vi "Execute Path with commands.vi"(0 "Iterations":i32, 1 "Sample Period":dbl, 2 "Commands":T2(array[cluster]) {"System" items=["Elevator", "Floating Intake", "Carriage Intake"]; "System Selection" items=["Elevator", "Floating Intake", "Carriage Intake"]}) -> ()   [LabVIEW 2018]
doc: "This VI notifies the subsystem to the new setpoint."
uses:
  Availible Command systems for auto.ctl
  <vilib>/Rock Robotics/WPI/Framework/Command Status Info.ctl
  <vilib>/Rock Robotics/WPI/Framework/Completion Status.ctl
  <vilib>/Rock Robotics/WPI/Framework/Completion Notifier.ctl
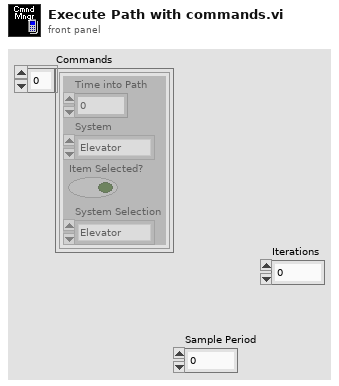
[diagram p1: front panel]
types:
  T1 = typedef "Availible Command systems for auto.ctl" = u16
  T2 = cluster{"Time into Path":dbl, "System":T1, "Item Selected?":bool, "System Selection":T1}[]
  T3 = cluster{"Time into Path":dbl, "System":T1, "Item Selected?":bool, "System Selection":T1}
  T4 = typedef "Command Status Info.ctl" = cluster{"Name":string, "Status":T5, "notifier out":T6}
  T5 = typedef "Completion Status.ctl" = enum16{"Successful", "Aborted", "Incomplete"}
  T6 = typedef "Completion Notifier.ctl" = refnum<notifier>
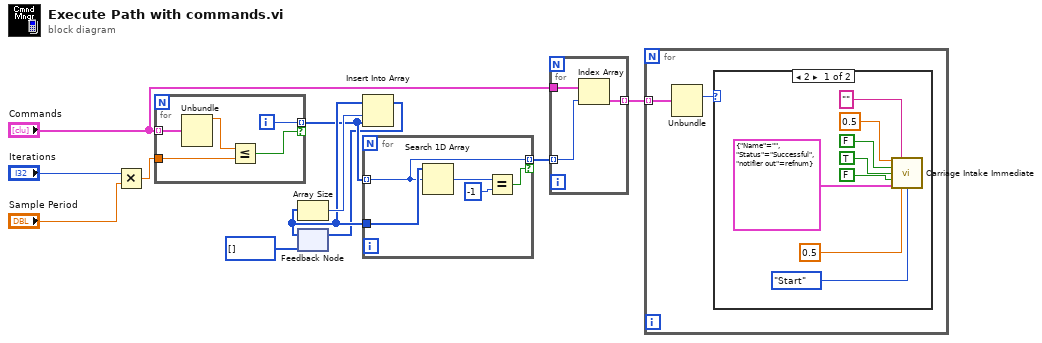
[diagram p0: block diagram]
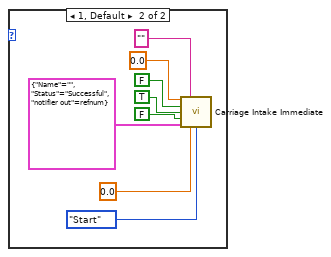
[diagram p2: hidden frame]
diagram:
  n1 = Multiply(x="Iterations", y="Sample Period") -> (x*y=w9:dbl)
  n2 = for {
    tunnel: "Commands" -> [w13] mode=indexing
    tunnel: w9 -> [w15]
    tunnel: [w12] -> w5 mode=indexing if=w14
    i -> [w12]
    n3 = Unbundle(w13) -> ("Time into Path"=w16:dbl)  [unwired: 3 out]
    n4 = Less Or Equal?(x=w16, y=w15) -> (x <= y?=w14:bool)
  }
  n5 = feedback #1(i32[] []) -> (w6:i32[])
  n6 = Array Size(array=w6) -> (size(s)=w7:i32)
  n7 = Insert Into Array(array=w6, index=w7, new element=w5) -> (w4:i32[])
  n8 = feedback-in #1(w4) -> ()
  n9 = for {
    tunnel: w6 -> [w21]
    tunnel: w5 -> [w18] mode=indexing
    tunnel: [w18] -> w2 mode=indexing if=w17
    n10 = Search 1D Array(1D array=w21, element=w18) -> (index of element=w20:i32)  [unwired: 1 in]
    n11 = Equal?(x=w20, y=-1) -> (x = y?=w17:bool)
  }
  n12 = for {
    tunnel: "Commands" -> [w24]
    tunnel: w2 -> [w23] mode=indexing
    tunnel: [w22] -> w1 mode=indexing
    n13 = Index Array(array=w24, index=w23) -> (element=w22:T3)
  }
  n14 = for {
    tunnel: w1 -> [w26] mode=indexing
    n15 = Unbundle(w26) -> ("System"=w25:T1)  [unwired: 3 out]
    n16 = case shown="2" w25 {
      frame 2 {
        n17 = call "Carriage Intake Immediate.vi"("Setpoint Left"=0.5, "Description"="", "Extend"=FALSE, "Open"=TRUE, "Close"=FALSE, "Command Info In"=T4 {"Name"="", "Status"=enum."Successful", "notifier out"=refnum}, "Setpoint Right"=0.5, "Synchronication"=enum16{"Start", "Wait"}."Start") -> ()  [unwired: 7 in, 1 out]
      }
      frame 1, Default {
        n18 = call "Carriage Intake Immediate.vi"("Setpoint Left"=0.0, "Description"="", "Extend"=FALSE, "Open"=TRUE, "Close"=FALSE, "Command Info In"=T4 {"Name"="", "Status"=enum."Successful", "notifier out"=refnum}, "Setpoint Right"=0.0, "Synchronication"=enum16{"Start", "Wait"}."Start") -> ()  [unwired: 7 in, 1 out]
      }
    }
  }
